vi "Pretty JSON.vi"(1 "JSON in":string) -> (0 "JSON out":string)   [LabVIEW 2018, in "CubeLogger.lvclass"]
uses:
  CubeLogger/CubeLogger.lvclass
  <vilib>/regexp/Match Regular Expression.xnode
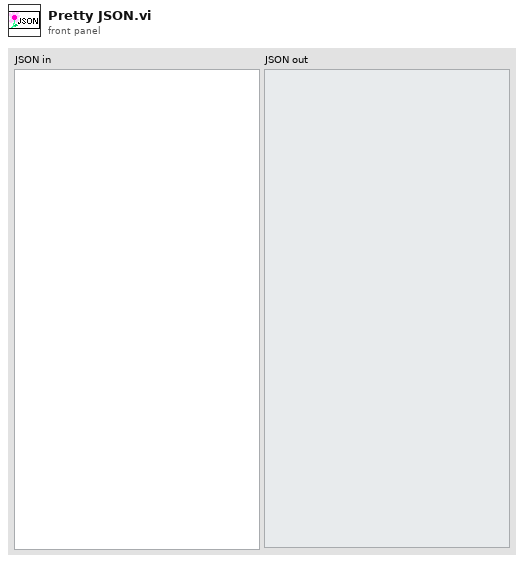
[diagram p1: front panel]
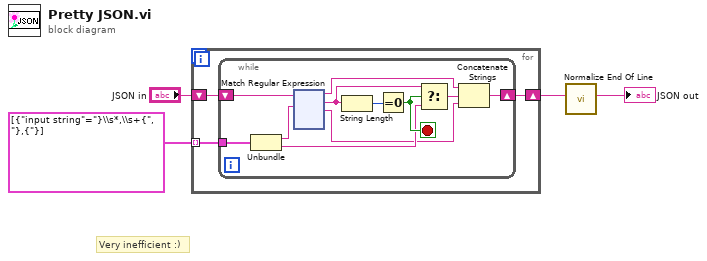
[diagram p0: block diagram]
diagram:
  # "Very inefficient :)"
  n1 = for {
    tunnel: cluster{"input string":string, string}[] [{"input string"="}\\s*,\\s+{", "},{"}] -> [w7] mode=indexing
    shift-right: [w5] -> w2
    shift-left: "JSON in" -> [w6]
    n2 = while {
      tunnel: w7 -> [w15]
      shift-right: [w8] -> w5
      shift-left: w6 -> [w13]
      stop <- w17 stop-if-true
      n3 = Unbundle(w15) -> ("input string"=w14:string, w12:string)
      n4 = xnode "Match Regular Expression"("input string"=w13, "regular expression"=w14) -> ("before match"=w11:string, "whole match"=w16:string, "after match"=w10:string)  [unwired: 4 in, 2 out]
      n5 = String Length(string=w16) -> (length=w18:i32)
      n6 = Equal To 0?(x=w18) -> (x = 0?=w17:bool)
      n7 = Select(t=w16, s=w17, f=w12) -> (s? t:f=w9:string)
      n8 = Concatenate Strings(w11, w9, w10) -> (w8:string)
    }
  }
  n9 = call <vilib>:"Normalize End Of Line.vi"("string in"=w2) -> ("string out"=→"JSON out":string)  [unwired: 7 in]
